vi "AO update.vi"(3 "device":i16=1, 4 "data":dbl[](array[numeric]) format="%0.4f") -> ()   [LabVIEW 2017]
uses:
  <vilib>/Utility/error.llb/DialogType.ctl
  <vilib>/DAQmx/write.llb/DAQmx Write (Analog 1D DBL NChan 1Samp).vi
  <vilib>/DAQmx/create/channels.llb/DAQmx Create Channel (AO-Voltage-Basic).vi
  <vilib>/DAQmx/configure/timing.llb/DAQmx Timing (Sample Clock).vi
  <vilib>/DAQmx/miscellaneous.llb/DAQmx Fill In Error Info.vi
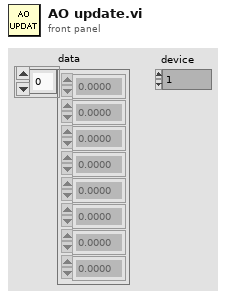
[diagram p1: front panel]
types:
  T1 = typedef "DialogType.ctl" = u16
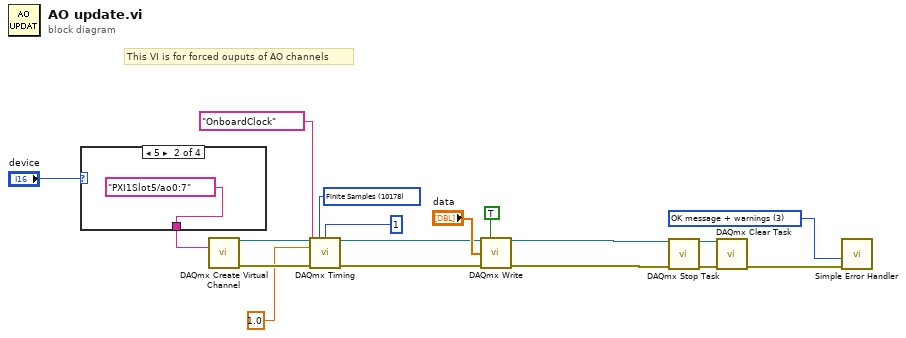
[diagram p0: block diagram]
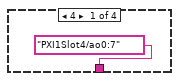
[diagram p2: hidden frame]
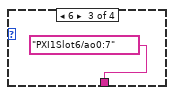
[diagram p3: hidden frame]
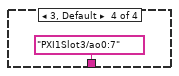
[diagram p4: hidden frame]
diagram:
  w12 = 10178 items=["Finite Samples"=10178, "Continuous Samples"=10123, "Hardware Timed Single Point"=12522] ("sample mode")
  w13 = T1 3 items=["no dialog", "OK message", "continue or stop message", "OK message + warnings", "continue/stop + warnings"] ("type of dialog (OK msg:1)")
  # "This VI is for forced ouputs of AO channels"
  n1 = case shown="5" "device" {
    tunnel: [tag "PXI1Slot4/ao0:7" ("physical channels") tag "PXI1Slot5/ao0:7" ("physical channels") tag "PXI1Slot6/ao0:7" ("physical channels") tag "PXI1Slot3/ao0:7" ("physical channels")] -> w10
    frame 4 {
    }
    frame 5 {
    }
    frame 6 {
    }
    frame 3, Default {
    }
  }
  n2 = call-poly <vilib>:"DAQmx Create Virtual Channel.vi"("physical channels"=w10) -> ("task out"=w17:refnum<k21>, "error out"=w18:errorcluster)  [unwired: 13 in]
  n3 = call-poly <vilib>:"DAQmx Timing.vi"("task/channels in"=w17, "sample mode"=w12, "samples per channel"=1, "rate"=1.0, "source"=tag "OnboardClock", "error in"=w18) -> ("task out"=w4:refnum<k21>, "error out"=w3:errorcluster)  [unwired: 8 in]
  n4 = call-poly <vilib>:"DAQmx Write.vi"("task/channels in"=w4, "auto start"=TRUE, "data"="data", "error in"=w3) -> ("task out"=w2:refnum<k21>, "error out"=w1:errorcluster)  [unwired: 9 in, 1 out]
  n5 = call <vilib>:"DAQmx Stop Task.vi"("task/channels in"=w2, "error in"=w1) -> ("task out"=w15:refnum<k21>, "error out"=w14:errorcluster)  [unwired: 12 in]
  n6 = call <vilib>:"DAQmx Clear Task.vi"("task in"=w15, "error in"=w14) -> ("error out"=w16:errorcluster)  [unwired: 13 in]
  n7 = call <vilib>:"Simple Error Handler.vi"("type of dialog (OK msg:1)"=w13, "error in (no error)"=w16) -> ()  [unwired: 3 in, 5 out]
